vi "Set Output.vi"(8 "error in (no error)":errorcluster, 10 "Enable":bool, 11 "Stanford Research PS350 in":refnum<class "Stanford Research PS350.lvclass">) -> (0 "error out":errorcluster, 3 "Stanford Research PS350 out":refnum<class "Stanford Research PS350.lvclass">)   [LabVIEW 2011, in "Stanford Research PS350.lvclass"]
uses:
  Stanford Research PS350.lvclass
  Stanford Research PS350.lvclass/Stanford Research PS350.ctl
  <instrlib>/Stanford Research PS300 Series/Stanford Research PS300 Series.lvlib
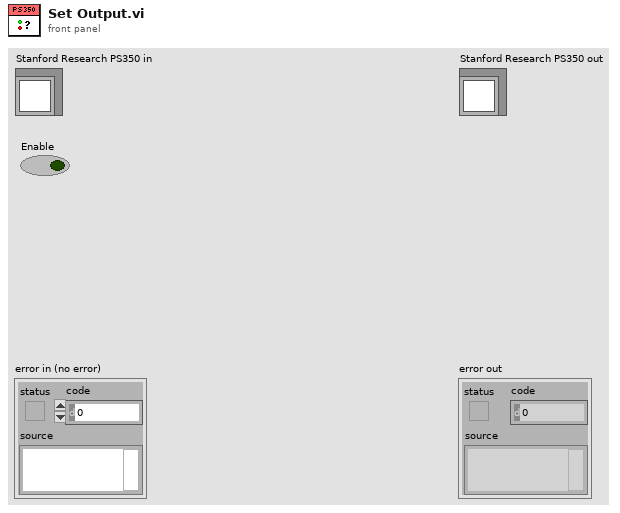
[diagram p1: front panel]
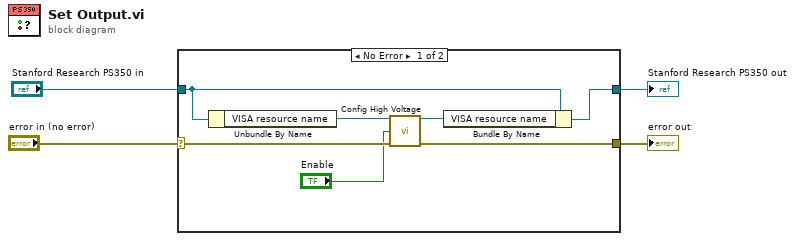
[diagram p0: block diagram]
diagram:
  n1 = case shown="No Error" "error in (no error)" {
    selector: "error in (no error)" -> [w7 w13]
    tunnel: [w6 w13] -> w3
    tunnel: [w10 w12] -> w1
    tunnel: "Stanford Research PS350 in" -> [w11 w12]
    frame No Error {
      n2 = Unbundle By Name(w11) -> ("VISA resource name"=w8:refnum<visa-resource-name>)
      n3 = call "Config High Voltage.vi"("VISA resource name"=w8, "High  Voltage Control (T:On)"="Enable", "error in (no error)"=w7) -> ("VISA resource name out"=w9:refnum<visa-resource-name>, "error out"=w6:errorcluster)  [unwired: 11 in]
      n4 = Bundle By Name(cluster=w11, "VISA resource name"=w9) -> (w10:refnum<class "Stanford Research PS350.lvclass">)
    }
    frame Error {
    }
  }
  "error out" <- w3
  "Stanford Research PS350 out" <- w1
